vi "Write Shaft Length.vi"(10 "length cm":dbl=100.0, 11 "Prybar in":refnum<class "Prybar.lvclass">) -> (3 "Prybar out":refnum<class "Prybar.lvclass">)   [LabVIEW 2023, in "Prybar.lvclass"]
uses:
  Prybar.lvclass
  Prybar.lvclass/Prybar.ctl
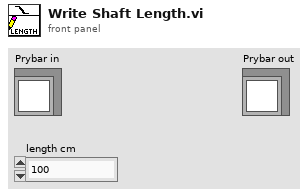
[diagram p1: front panel]
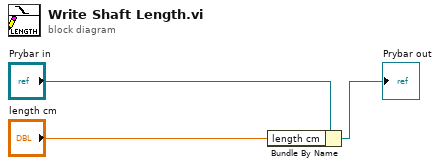
[diagram p0: block diagram]
diagram:
  n1 = Bundle By Name(cluster="Prybar in", "length cm"="length cm") -> (→"Prybar out":refnum<class "Prybar.lvclass">)
